vi "Test_WriteValue_ActorDead_ReturnError.vi"(8 "error in (no error)":errorcluster, 11 "TestCase in":refnum<class "TestActorMessageTransport.lvclass">) -> (0 "error out":errorcluster, 3 "TestCase out":refnum<class "TestActorMessageTransport.lvclass">)   [LabVIEW 2017, in "TestActorMessageTransport.lvclass"]
uses:
  TestActorMessageTransport.lvclass
  <vilib>/ActorFramework/Actor/Actor.lvclass
  MockNotificationMsg/MockNotificationMsg.lvclass/MockNotificationMsg.ctl
  <vilib>/ActorFramework/Message Enqueuer/Message Enqueuer.lvclass/Message Enqueuer.ctl
  Source/Concrete/ActorMessageTransport/ActorMessageTransport.lvclass/ActorMessageTransport.ctl
  <vilib>/ActorFramework/Message Enqueuer/Enqueue.vi
  <vilib>/ActorFramework/Message Enqueuer/Equals Not A Refnum.vi
  MockNotificationMsg/MockNotificationMsg.lvclass
  C:/Git/composed-transport/Source/Concrete/ActorMessageTransport/Notification Msg/Notification Msg.lvclass
  Source/Concrete/ActorMessageTransport/ActorMessageTransport.lvclass
  C:/Git/composed-transport/Source/ITransport/ITransport.lvclass
  <vilib>/ActorFramework/Stop Msg/Stop Msg.lvclass
  C:/Program Files (x86)/National Instruments/LabVIEW 2017/vi.lib/ActorFramework/Message/Message.lvclass
  <vilib>/Utility/error.llb/Error Cluster From Error Code.vi
  <vilib>/ActorFramework/Message Priority Queue/Priority Enqueue.vi
  <vilib>/ActorFramework/Message Enqueuer/Message Enqueuer.lvclass
  Source/Concrete/ActorMessageTransport/Notification Msg/Notification Msg.lvclass
  Source/ITransport/ITransport.lvclass
panel:
  out "Return Error":errorcluster
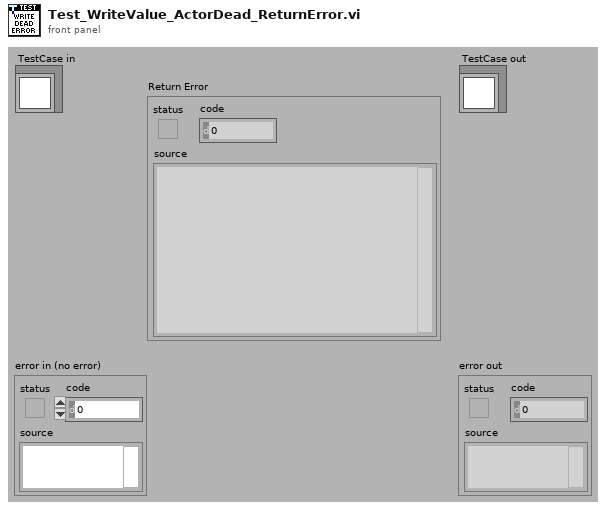
[diagram p1: front panel]
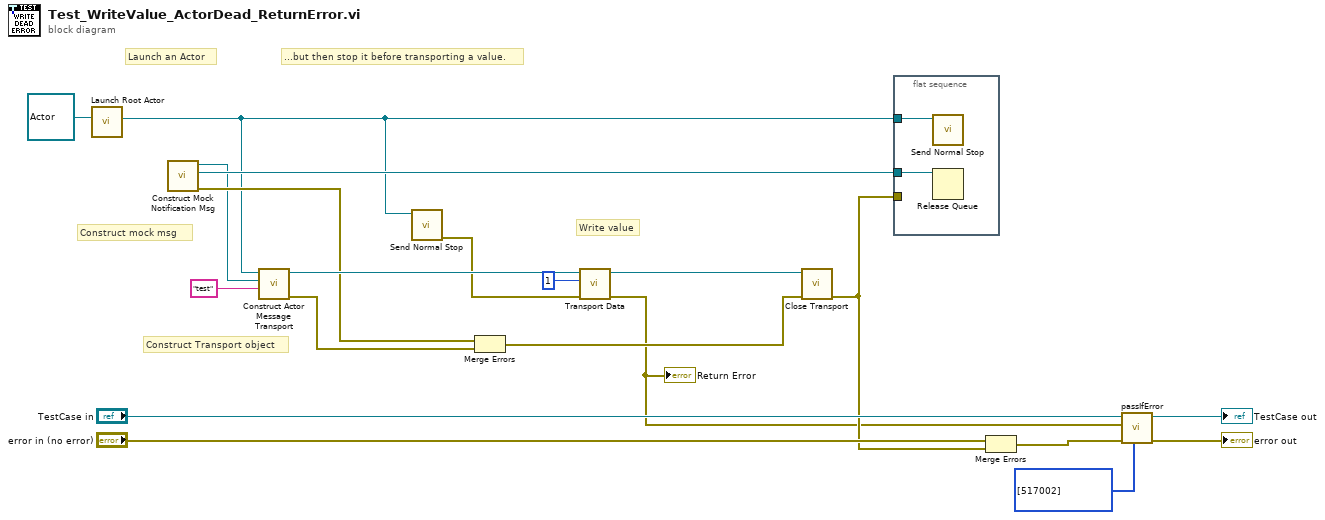
[diagram p0: block diagram]
diagram:
  # "...but then stop it before transporting a value."
  # "Launch an Actor"
  # "Construct Transport object"
  # "Construct mock msg"
  # "Write value"
  n1 = call <vilib>:"Launch Root Actor.vi"("Actor"=refnum<class "Actor.lvclass"> refnum) -> ("Actor's Enqueuer"=w2:refnum<class "Message Enqueuer.lvclass">)  [unwired: 9 in, 1 out]
  n2 = call "Construct Mock Notification Msg.vi"() -> ("error out"=w19:errorcluster, "Data leak test queue"=w10:refnum<queue>, "MockNotificationMsg out"=w8:refnum<class "MockNotificationMsg.lvclass">)  [unwired: 9 in]
  n3 = call "Construct Actor Message Transport.vi"("Datum Name"="test", "Notification Msg"=w8, "Message Enqueuer in"=w2) -> ("error out"=w13:errorcluster, "ActorMessageTransport"=w20:refnum<class "ActorMessageTransport.lvclass">)  [unwired: 7 in]
  n4 = call <vilib>:"Send Normal Stop.vi"("Message Enqueuer"=w2) -> ("error out"=w1:errorcluster)  [unwired: 10 in]
  n5 = Merge Errors(w19, w13) -> (w6:errorcluster)
  n6 = call "Transport Data.vi"("error in (no error)"=w1, "Value"=1, "ITransport in"=w20) -> ("error out"=w5:errorcluster, "ITransport out"=w12:refnum<class "ActorMessageTransport.lvclass">)  [unwired: 7 in]
  "Return Error" <- w5
  n7 = call-dynamic "Close Transport.vi"("error in (no error)"=w6, "ITransport in"=w12) -> ("error out"=w9:errorcluster)  [unwired: 9 in]
  n8 = flat-sequence {
    tunnel: w10 -> [w22]
    tunnel: w2 -> [w21]
    tunnel: w9 -> [_]
    frame #0 {
      n9 = call <vilib>:"Send Normal Stop.vi"("Message Enqueuer"=w21) -> ()  [unwired: 10 in, 1 out]
      n10 = Release Queue(queue=w22) -> ()  [unwired: 2 in, 3 out]
    }
  }
  n11 = Merge Errors("error in (no error)", w9) -> (w14:errorcluster)
  n12 = call-dynamic "passIfError.vi"("passing error codes (default = any error code)"=i32[] [517002], "error in (no error)"=w14, "error"=w5, "TestCase in"="TestCase in") -> ("error out"=→"error out":errorcluster, "TestCase out"=→"TestCase out":refnum<class "TestActorMessageTransport.lvclass">)  [unwired: 6 in]
